vi "Map Master AO to Slave AI for Fixture T-801.vi"(10 "slave device":string="DAQ2", 11 "AO Write Channels (Master)":string[](array[string])=["Targets/Controller/Hardware/Chassis/DAQ/DAQ1/Analog Output/AO0", "Targets/Controller/Hardware/Chassis/DAQ/DAQ1/Analog Output/AO1"]) -> (3 "Map from AO Master to AI Slave":map{string, string[]}(c390))   [LabVIEW 2020, in "VeriStandTestCase.lvclass"]
doc: "Maps Master AO channels to Slave AI channels for connections made with the T-801 test fixture."
uses:
  VeriStandTestCase.lvclass
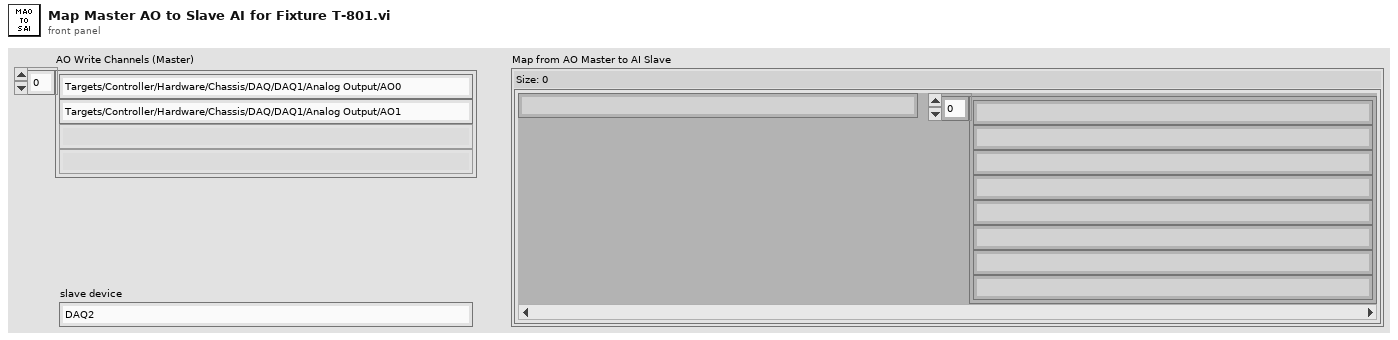
[diagram p1: front panel]
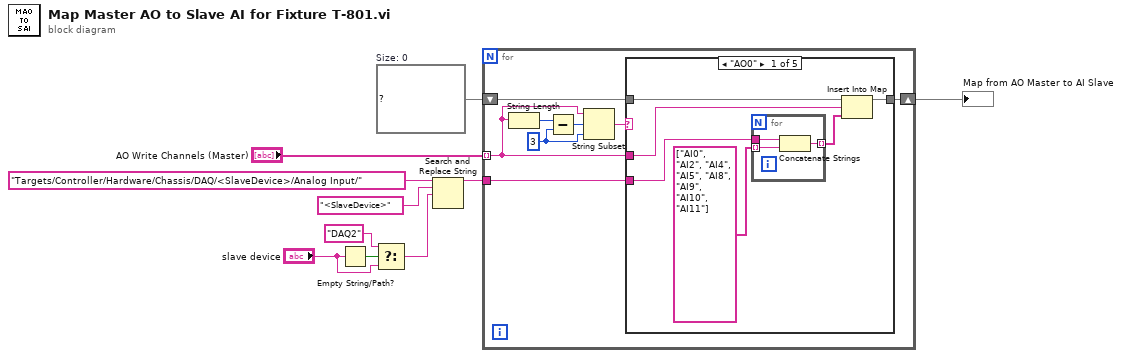
[diagram p0: block diagram]
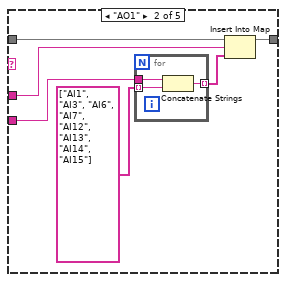
[diagram p2: hidden frame]
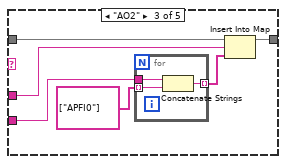
[diagram p3: hidden frame]
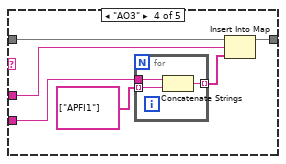
[diagram p4: hidden frame]
diagram:
  w3 = map{string, string[]} {}  # Size: 0
  n1 = Empty String/Path?(string/path="slave device") -> (empty?=w10:bool)
  n2 = Select(t="DAQ2", s=w10, f="slave device") -> (s? t:f=w5:string)
  n3 = Search and Replace String(input string="Targets/Controller/Hardware/Chassis/DAQ/<SlaveDevice>/Analog Input/", search string="<SlaveDevice>" ("substring (\"\")"), replace string=w5) -> (result string=w2:string)  [unwired: 5 in, 3 out]
  n4 = for {
    tunnel: "AO Write Channels (Master)" -> [w12] mode=indexing
    tunnel: w2 -> [w17]
    shift-right: [w16] -> w1
    shift-left: w3 -> [w18]
    w11 = 3 ("length (rest)")
    n5 = String Length(string=w12) -> (length=w15:i32)
    n6 = Subtract(x=w15, y=w11) -> (x-y=w14:i32)
    n7 = String Subset(string=w12, offset (0)=w14, length (rest)=w11) -> (substring=w13:string)
    n8 = case shown="\"AO0\"" w13 {
      tunnel: w12 -> [w23 w32 w41 w50 _]
      tunnel: w18 -> [w24 w33 w42 w51 w55]
      tunnel: w17 -> [w21 w31 w40 w49 _]
      tunnel: [w19 w28 w37 w46 w55] -> w16
      frame "AO0" {
        n9 = for {
          tunnel: string[] ["AI0", "AI2", "AI4", "AI5", "AI8", "AI9", "AI10", "AI11"] -> [w27] mode=indexing
          tunnel: w21 -> [w26]
          tunnel: [w25] -> w20 mode=indexing
          n10 = Concatenate Strings(w26, w27) -> (w25:string)
        }
        n11 = Insert Into Map(map in=w24, key=w23, value=w20) -> (map out=w19:map{string, string[]})  [unwired: 2 out]
      }
      frame "AO1" {
        n12 = for {
          tunnel: string[] ["AI1", "AI3", "AI6", "AI7", "AI12", "AI13", "AI14", "AI15"] -> [w36] mode=indexing
          tunnel: w31 -> [w35]
          tunnel: [w34] -> w30 mode=indexing
          n13 = Concatenate Strings(w35, w36) -> (w34:string)
        }
        n14 = Insert Into Map(map in=w33, key=w32, value=w30) -> (map out=w28:map{string, string[]})  [unwired: 2 out]
      }
      frame "AO2" {
        n15 = for {
          tunnel: string[] ["APFI0"] -> [w45] mode=indexing
          tunnel: w40 -> [w44]
          tunnel: [w43] -> w39 mode=indexing
          n16 = Concatenate Strings(w44, w45) -> (w43:string)
        }
        n17 = Insert Into Map(map in=w42, key=w41, value=w39) -> (map out=w37:map{string, string[]})  [unwired: 2 out]
      }
      frame "AO3" {
        n18 = for {
          tunnel: string[] ["APFI1"] -> [w54] mode=indexing
          tunnel: w49 -> [w53]
          tunnel: [w52] -> w48 mode=indexing
          n19 = Concatenate Strings(w53, w54) -> (w52:string)
        }
        n20 = Insert Into Map(map in=w51, key=w50, value=w48) -> (map out=w46:map{string, string[]})  [unwired: 2 out]
      }
      frame Default {
      }
    }
  }
  "Map from AO Master to AI Slave" <- w1
